vi "aryapp.vi"() -> ()   [LabVIEW 2022 SP3]
panel:
  in  "右":bool
  in  "左":bool
  in  "上":bool
  in  "下":bool
  in  "Stop":bool
  in  "列":dbl
  in  "行":dbl
  out "Current Position Array":bool[][](array[boolean])=[[TRUE, TRUE, TRUE], [TRUE, FALSE, TRUE], [TRUE, TRUE, TRUE]]
  out "Boolean":bool=TRUE
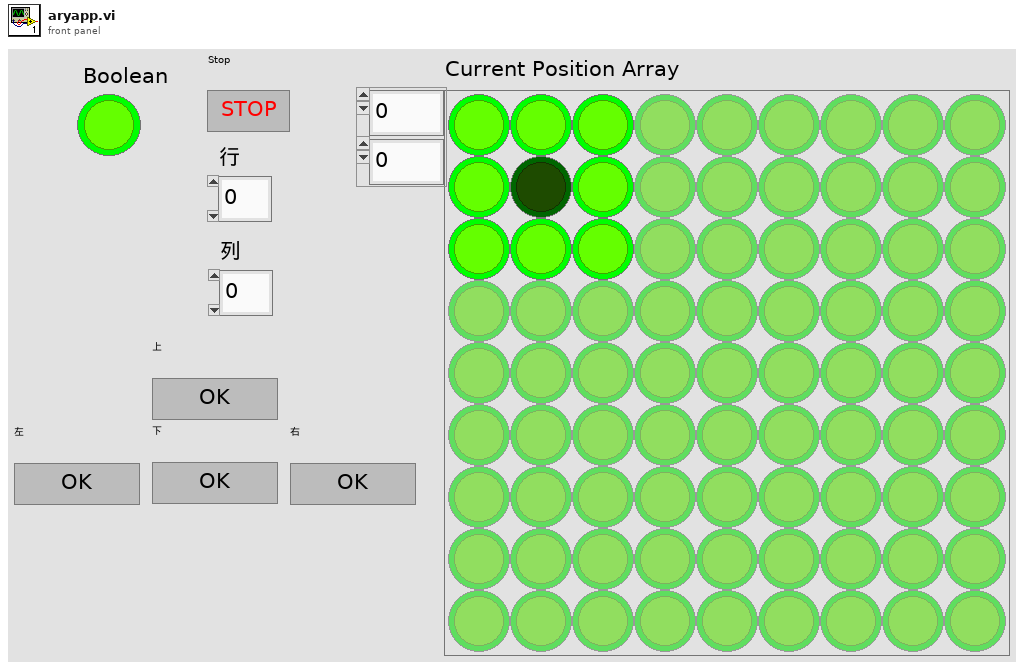
[diagram p1: front panel]
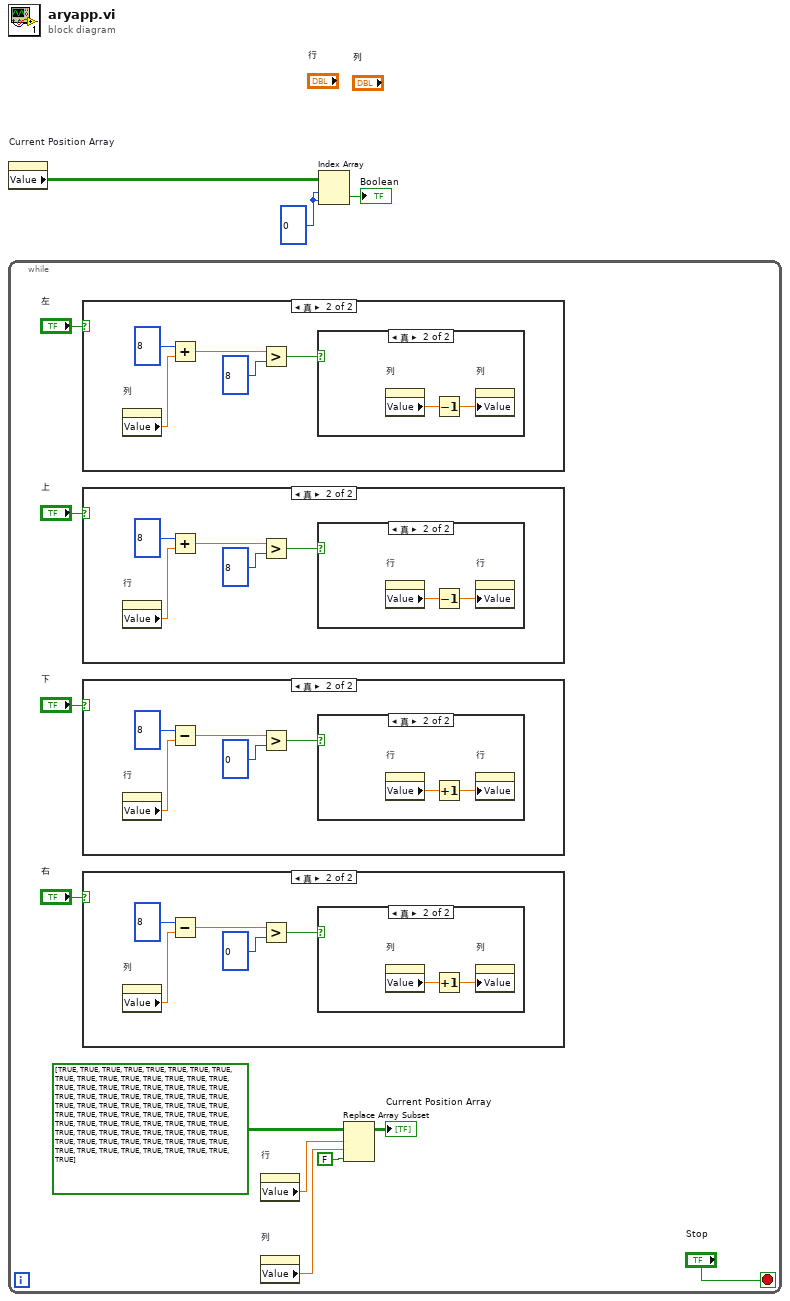
[diagram p0: block diagram]
diagram:
  w3 = 0
  n1 = property on="Current Position Array" class="Arr (严格)"() -> ("Value"=w1:bool[][])  [unwired: 2 in, 2 out]
  n2 = while {
    stop <- "Stop" stop-if-true
    n3 = case shown="真" "左" {
      frame False {
      }
      frame True {
        n4 = property on="列" class="DigNum (严格)"() -> ("Value"=w21:dbl)  [unwired: 2 in, 2 out]
        n5 = Add(x=8, y=w21) -> (x+y=w23:dbl)
        n6 = Greater?(x=w23, y=8) -> (0:w24:bool)
        n7 = case shown="真" w24 {
          frame False {
          }
          frame True {
            n8 = property on="列" class="DigNum (严格)"() -> ("Value"=w27:dbl)  [unwired: 2 in, 2 out]
            n9 = Decrement(x=w27) -> (x-1=w26:dbl)
            n10 = property on="列" class="DigNum (严格)"("Value"=w26) -> ()  [unwired: 2 in, 2 out]
          }
        }
      }
    }
    n11 = case shown="真" "上" {
      frame False {
      }
      frame True {
        n12 = property on="行" class="DigNum (严格)"() -> ("Value"=w28:dbl)  [unwired: 2 in, 2 out]
        n13 = Add(x=8, y=w28) -> (x+y=w30:dbl)
        n14 = Greater?(x=w30, y=8) -> (0:w31:bool)
        n15 = case shown="真" w31 {
          frame False {
          }
          frame True {
            n16 = property on="行" class="DigNum (严格)"() -> ("Value"=w34:dbl)  [unwired: 2 in, 2 out]
            n17 = Decrement(x=w34) -> (x-1=w33:dbl)
            n18 = property on="行" class="DigNum (严格)"("Value"=w33) -> ()  [unwired: 2 in, 2 out]
          }
        }
      }
    }
    n19 = case shown="真" "下" {
      frame False {
      }
      frame True {
        n20 = property on="行" class="DigNum (严格)"() -> ("Value"=w35:dbl)  [unwired: 2 in, 2 out]
        n21 = Subtract(x=8, y=w35) -> (x-y=w37:dbl)
        n22 = Greater?(x=w37, y=0) -> (0:w38:bool)
        n23 = case shown="真" w38 {
          frame False {
          }
          frame True {
            n24 = property on="行" class="DigNum (严格)"() -> ("Value"=w41:dbl)  [unwired: 2 in, 2 out]
            n25 = Increment(x=w41) -> (x+1=w40:dbl)
            n26 = property on="行" class="DigNum (严格)"("Value"=w40) -> ()  [unwired: 2 in, 2 out]
          }
        }
      }
    }
    n27 = case shown="真" "右" {
      frame False {
      }
      frame True {
        n28 = property on="列" class="DigNum (严格)"() -> ("Value"=w14:dbl)  [unwired: 2 in, 2 out]
        n29 = Subtract(x=8, y=w14) -> (x-y=w16:dbl)
        n30 = Greater?(x=w16, y=0) -> (0:w17:bool)
        n31 = case shown="真" w17 {
          frame False {
          }
          frame True {
            n32 = property on="列" class="DigNum (严格)"() -> ("Value"=w20:dbl)  [unwired: 2 in, 2 out]
            n33 = Increment(x=w20) -> (x+1=w19:dbl)
            n34 = property on="列" class="DigNum (严格)"("Value"=w19) -> ()  [unwired: 2 in, 2 out]
          }
        }
      }
    }
    n35 = property on="行" class="DigNum (严格)"() -> ("Value"=w10:dbl)  [unwired: 2 in, 2 out]
    n36 = property on="列" class="DigNum (严格)"() -> ("Value"=w9:dbl)  [unwired: 2 in, 2 out]
    n37 = Replace Array Subset(array=bool[][] [[TRUE, TRUE, TRUE, TRUE, TRUE, TRUE, TRUE, TRUE, TRUE], [TRUE, TRUE, TRUE, TRUE, TRUE, TRUE, TRUE, TRUE, TRUE], [TRUE, TRUE, TRUE, TRUE, TRUE, TRUE, TRUE, TRUE, TRUE], [TRUE, TRUE, TRUE, TRUE, TRUE, TRUE, TRUE, TRUE, TRUE], [TRUE, TRUE, TRUE, TRUE, TRUE, TRUE, TRUE, TRUE, TRUE], [TRUE, TRUE, TRUE, TRUE, TRUE, TRUE, TRUE, TRUE, TRUE], [TRUE, TRUE, TRUE, TRUE, TRUE, TRUE, TRUE, TRUE, TRUE], [TRUE, TRUE, TRUE, TRUE, TRUE, TRUE, TRUE, TRUE, TRUE], [TRUE, TRUE, TRUE, TRUE, TRUE, TRUE, TRUE, TRUE, TRUE]], new element=FALSE, index (row)=w10, index (col)=w9) -> (→"Current Position Array":bool[][])
  }
  n38 = Index Array(array=w1, index (row)=w3, index (col)=w3) -> (element=→"Boolean":bool)
